vi "Calc Target Voltages Step 1.vi"(10 "output cluster":T1) -> ()   [LabVIEW 2016]
uses:
  Controls/Cal Refs.ctl
  <vilib>/Analysis/baseanly.llb/Mean (DBL).vi
  Miscellaneous/Globals.vi
  <vilib>/Analysis/NI_AALBase.lvlib
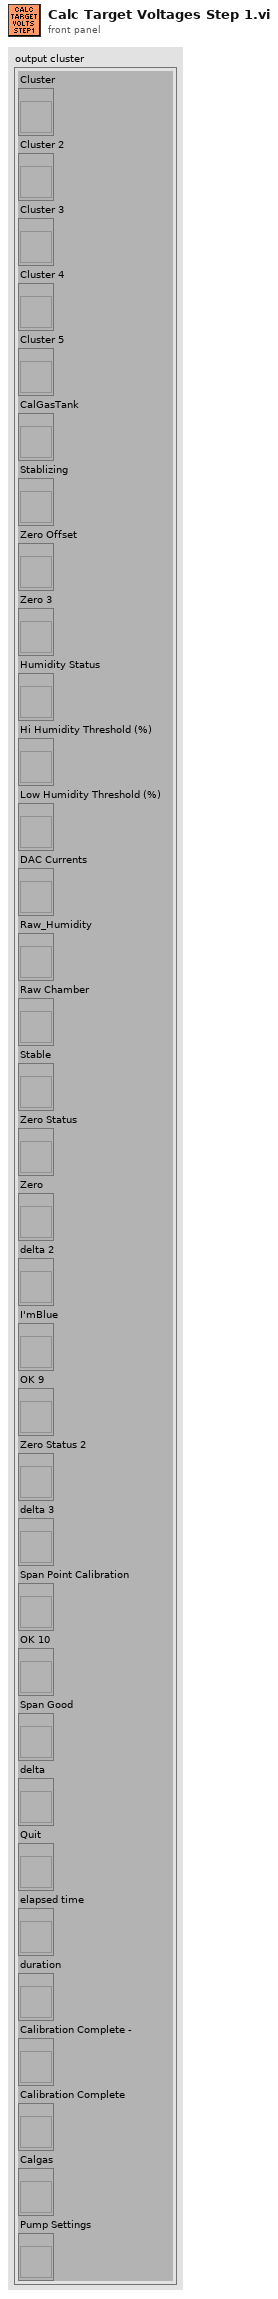
[diagram p1: front panel]
types:
  T1 = typedef "Cal Refs.ctl" = cluster{"Cluster":refnum<vi>, "Cluster 2":refnum<vi>, "Cluster 3":refnum<vi>, "Cluster 4":refnum<vi>, "Cluster 5":refnum<vi>, "CalGasTank":refnum<vi>, "Stablizing":refnum<vi>, "Zero Offset":refnum<vi>, "Zero 3":refnum<vi>, "Humidity Status":refnum<vi>, "Hi Humidity Threshold (%)":refnum<vi>, "Low Humidity Threshold (%)":refnum<vi>, "DAC Currents":refnum<vi>, "Raw_Humidity":refnum<vi>, "Raw Chamber":refnum<vi>, "Stable":refnum<vi>, "Zero Status":refnum<vi>, "Zero":refnum<vi>, "delta 2":refnum<vi>, "I'mBlue":refnum<vi>, "OK 9":refnum<vi>, "Zero Status 2":refnum<vi>, "delta 3":refnum<vi>, "Span Point Calibration":refnum<vi>, "OK 10":refnum<vi>, "Span Good":refnum<vi>, "delta":refnum<vi>, "Quit":refnum<vi>, "elapsed time":refnum<vi>, "duration":refnum<vi>, "Calibration Complete -":refnum<vi>, "Calibration Complete":refnum<vi>, "Calgas":refnum<vi>, "Pump Settings":refnum<vi>}
  T2 = cluster{"Tcal_Chamber":dbl, "Tcal_PCB":dbl, "Tcal_Film":dbl, "Tcal_Humidity":dbl, "Tcal_Det":dbl[], "Cal Gas":dbl, "Reference":dbl}
  T3 = typedef "Calibration Coefficients.ctl" = cluster{"CalFile Used":path, "TYPE":string, "DATE":string, "Humidity":sgl, "Chamber Temp":dbl, "CO2_calgas":dbl, "V_(RA,5mA)":dbl, "V_(RA,15mA)":dbl, "mI":dbl, "V_0d_ImA (actual)":dbl, "V_6d_ImA (actual)":dbl, "I_span":dbl, "DAC":u16, "A":dbl, "B":dbl, "C":dbl, "D":dbl, "V6d":dbl, "A'":dbl, "B'":dbl, "C'":dbl, "D'":dbl, "V0d":dbl, "CalDate":string, "CalTime":string, "duration":dbl, "Detector Channel":string, "a2":dbl, "a3":dbl, "a4":dbl, "a5":dbl, "b2":dbl, "c2":dbl, "b3":dbl, "c3":dbl, "b4":dbl, "c4":dbl, "b5":dbl, "c5":dbl, "a7":dbl, "a8":dbl, "a9":dbl, "a10":dbl, "b7":dbl, "b8":dbl, "b9":dbl, "b10":dbl, "c7":dbl, "c8":dbl, "c9":dbl, "c10":dbl, "cal_offs_adj":dbl, "cal_gain_adj":dbl, "C6d":dbl, "C0d":dbl, "Cal_currernt":dbl, "C2V":u16, "V2C":u16, "Zero Date":string, "Zero Time":string, "Number of Zeroes":u16, "V_(()d, average)":dbl, "V_offs ":dbl, "G_adj":dbl, "Pump Flow Rate":u16, "Zero Required? ":bool, "Calibrate Required?":bool, "cal_utc":dbl, "zero_utc":dbl, "Elapsed Time":dbl, "PCB":string, "m0":dbl, "b0":dbl}
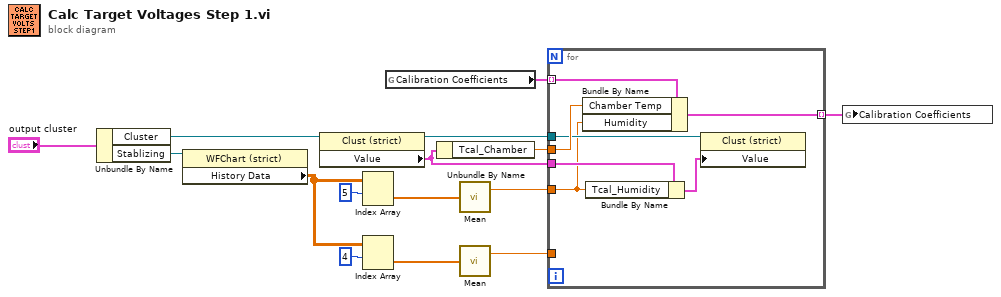
[diagram p0: block diagram]
diagram:
  n1 = Unbundle By Name("output cluster") -> ("Cluster"=w15:refnum<vi>, "Stablizing"=w3:refnum<vi>)
  n2 = property on="Property Node" class="WFChart (strict)"(reference=w3) -> ("History Data"=w8:dbl[][])  [unwired: 1 in, 2 out]
  n3 = property class="Clust (strict)"(reference=w15) -> (reference out=w13:refnum<vi>, "Value"=w12:T2)  [unwired: 1 in, 1 out]
  n4 = Index Array(array=w8, index (row)=5) -> (element=w6:dbl[])  [unwired: 1 in]
  n5 = Index Array(array=w8, index (row)=4) -> (element=w5:dbl[])  [unwired: 1 in]
  n6 = global read "Globals.vi" "Calibration Coefficients"() -> (w2:T3[])
  n7 = Unbundle By Name(w12) -> ("Tcal_Chamber"=w11:dbl)
  n8 = call-poly <vilib>:"Mean.vi"("X"=w6) -> ("mean"=w10:dbl)  [unwired: 1 out]
  n9 = call-poly <vilib>:"Mean.vi"("X"=w5) -> ("mean"=w9:dbl)  [unwired: 1 out]
  n10 = for {
    tunnel: w9 -> [_]
    tunnel: [w22] -> w1 mode=indexing
    tunnel: w10 -> [w16]
    tunnel: w2 -> [w21] mode=indexing
    tunnel: w11 -> [w20]
    tunnel: w12 -> [w19]
    tunnel: w13 -> [w17]
    n11 = Bundle By Name(cluster=w21, "Chamber Temp"=w20, "Humidity"=w16) -> (w22:T3)
    n12 = Bundle By Name(cluster=w19, "Tcal_Humidity"=w16) -> (w18:T2)
    n13 = property class="Clust (strict)"(reference=w17, "Value"=w18) -> ()  [unwired: 1 in, 2 out]
  }
  n14 = global write "Globals.vi" "Calibration Coefficients"(w1) -> ()
